vi "Drive Execute.vi"() -> ()   [LabVIEW 2017]
uses:
  Drive Control Type.ctl
  <vilib>/Rock Robotics/WPI/Solenoid/WPI_SolenoidValue.ctl
  <vilib>/Rock Robotics/WPI/DriverStation/WPI_DriverStationRobotMode2.ctl
  Drive Notifier.ctl
  <vilib>/Rock Robotics/WPI/ThirdParty/Phoenix-LabVIEW/Motor Controller/Controls/CTRE_Phoenix_MotorControl_ControlMode.ctl
  Drive Globals.vi
  Utility VIs/Refnum Names.vi
  Robot Global Data.vi
  <vilib>/Rock Robotics/WPI/Solenoid/WPI_SolenoidSetEnum.vi
  Autonomous/Autonomous Globals.vi
panel:
  out "Drive Motor Speeds-Teleop":T1(graph)
  out "error out":errorcluster
  in  "Maximum Low Linear Speed":dbl=5.49
  in  "Maximum High Linear Speed":dbl
  in  "Lower Multiplier":dbl=0.4
  in  "Upper Multiplier":dbl=0.65
  in  "Piecewise Turn Threshold":dbl=0.4
  in  "Lower Turn Speed":dbl=3.0
  in  "Upper Turn Speed":dbl=7.0
  in  "Scale Intertia":dbl=0.75
  # "Turning to Cube"
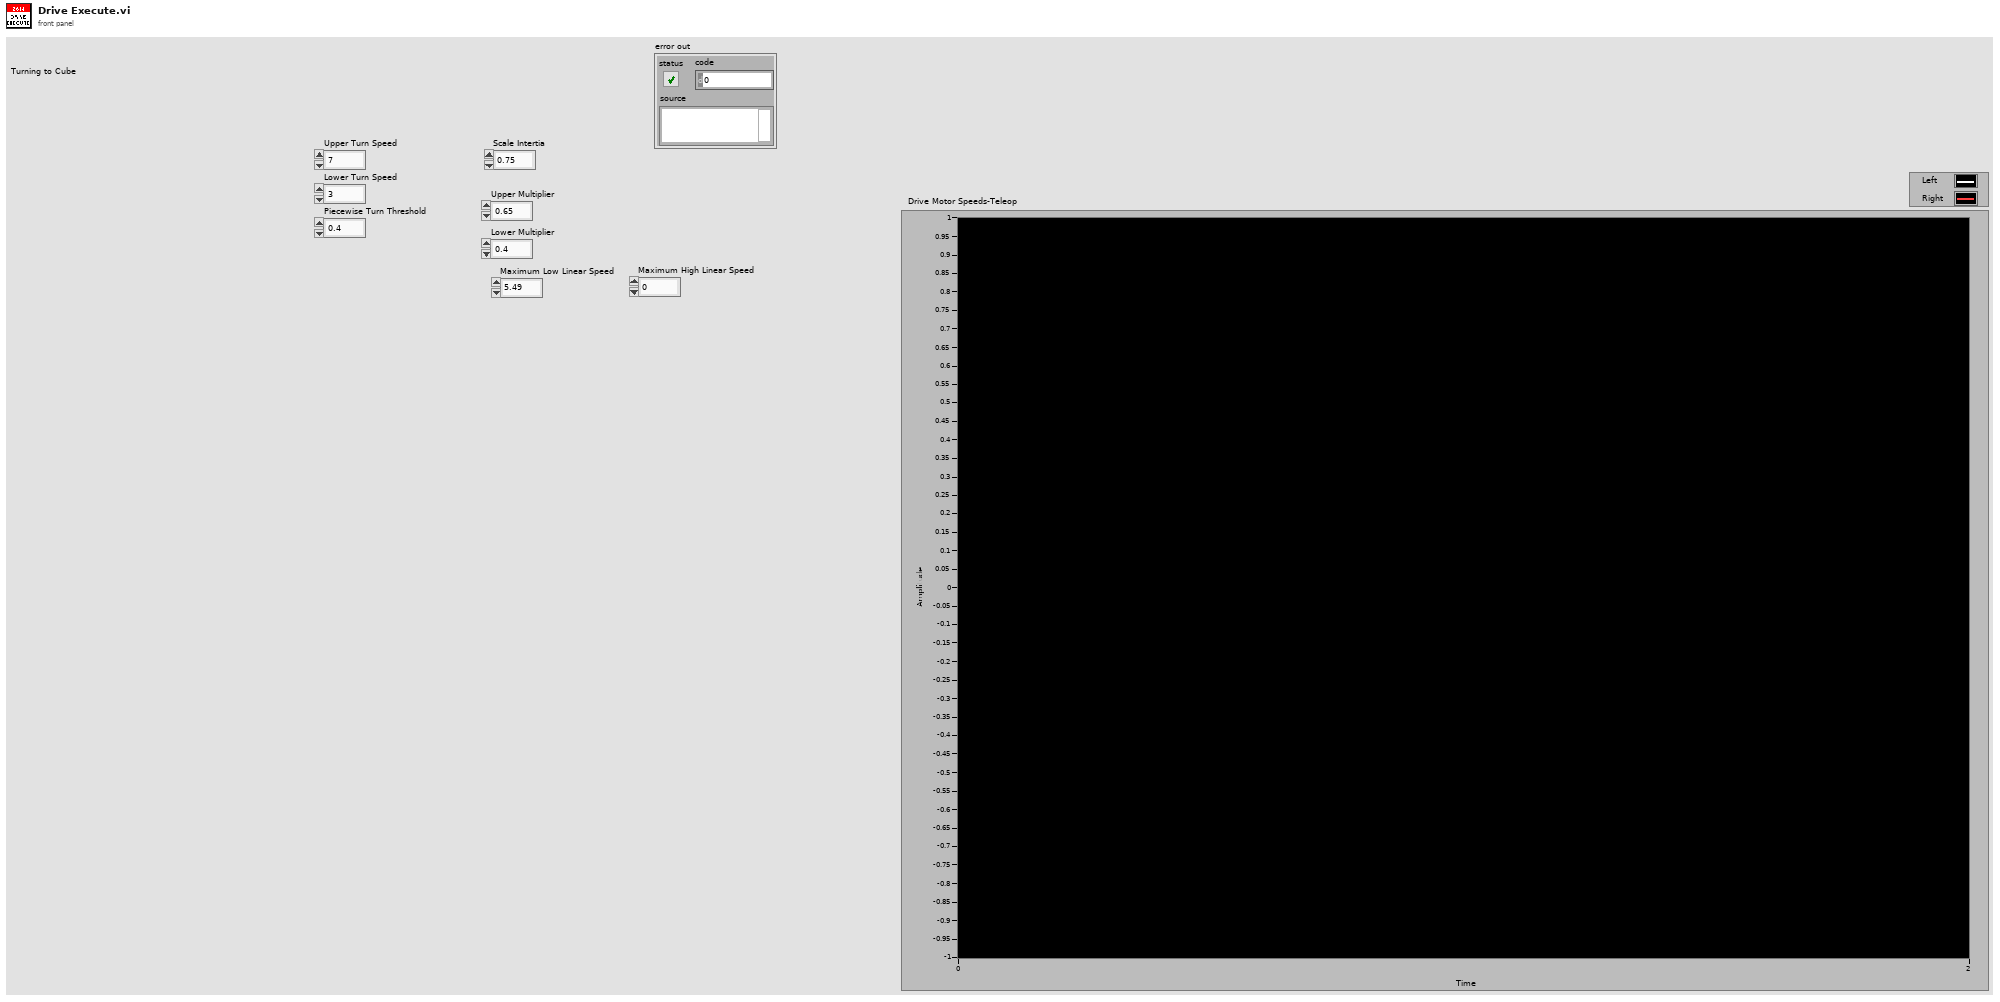
[diagram p1: front panel]
types:
  T1 = cluster{"Velocity (Raw Sensor Units per 100 ms)":i32, "Velocity (Raw Sensor Units per 100 ms)":i32, "Left Motor Value":dbl, dbl}
  T2 = typedef "WPI_MotorControlDeviceRef.ctl" = cluster{"DeviceStatus":errorcluster, "Type":T3, "PWM":cluster{"PWM Channel":T4, "DeadBand":T5}, "CAN":cluster{"Device Number":u8, "SetOutput VI Ref":variant, "GetOutput VI Ref":variant, "Enable VI Ref":variant, "Disable VI Ref":variant, "Data":variant}, "Invert":bool, "DIO PWM":cluster{"PWM \"Enable\" Channel":T4, "DIOChannel":T6, "PWM Rate":dbl}}
  T3 = typedef "WPI_MotorControlType.ctl" = enum16{"PWM", "CAN", "DIO PWM"}
  T4 = typedef "FPGA_DIOPWMChannel.ctl" = enum8{"PWM 0", "PWM 1", "PWM 2", "PWM 3", "PWM 4", "PWM 5", "PWM 6", "PWM 7", "PWM 8", "PWM 9", "PWM MXP 0", "PWM MXP 1", "PWM MXP 2", "PWM MXP 3", "PWM MXP 4", "PWM MXP 5", "PWM MXP 6", "PWM MXP 7", "PWM MXP 8", "PWM MXP 9", "Invalid"}
  T5 = typedef "WPI_PWMDeadband.ctl" = cluster{"Name":string, "maxPositivePwm":i32, "minPositivePwm":i32, "centerPwm":i32, "maxNegativePwm":i32, "minNegativePwm":i32, "angularRange":u16}
  T6 = typedef "FPGA_DIOChannel.ctl" = enum8{"DIO 0", "DIO 1", "DIO 2", "DIO 3", "DIO 4", "DIO 5", "DIO 6", "DIO 7", "DIO 8", "DIO 9", "DIO MXP 0", "DIO MXP 1", "DIO MXP 2", "DIO MXP 3", "DIO MXP 4", "DIO MXP 5", "DIO MXP 6", "DIO MXP 7", "DIO MXP 8", "DIO MXP 9", "DIO MXP 10", "DIO MXP 11", "DIO MXP 12", "DIO MXP 13", "DIO MXP 14", "DIO MXP 15", "SPI Port CS1", "SPI Port CS2", "SPI Port CS3", "SPI Port MISO", "SPI Port MOSI", "Invalid"}
  T7 = typedef "WPI_SolenoidDevRef.ctl" = cluster{"DevStatus":errorcluster, "Pneumatics Control Module":u8, "Forward Solenoid Channel":T8, "Reverse Solenoid Channel":T8}
  T8 = typedef "WPI_SolenoidChannel.ctl" = enum8{"Solenoid 0", "Solenoid 1", "Solenoid 2", "Solenoid 3", "Solenoid 4", "Solenoid 5", "Solenoid 6", "Solenoid 7", "Invalid"}
  T9 = typedef "WPI_SolenoidValue.ctl" = enum16{"Off", "On", "Forward", "Reverse"}
  T10 = typedef "Drive Control Type.ctl" = enum16{"No_Op", "Basic Drive", "Time", "Heading", "Hybrid_Turn", "RC_Speed", "Switch_Slots", "AutoTrack_Cube", "Speed Test", "Turn_Cube", "To_Cube", "Wait", "Distance_Slow", "Distance", "D_H_Delay", "Distance_Delay", "Heading_Cap", "Heading_Tight", "Cube_Heading", "Distance_Ramp"}
  T11 = typedef "WPI_DriverStationRobotMode2.ctl" = enum16{"Autonomous Disabled", "Autonomous Enabled", "Teleop Disabled", "Teleop Enabled", "Disconnected", "Finish", "Test Disabled", "Test Enabled", "Emergency Stopped"}
  T12 = typedef "Drive Notifier.ctl" = cluster{"Drive Control Type":T10, "Throttle":dbl, "Twist":dbl, "Step":i32, "High Gear":bool, "Parameter 1":dbl, "Parameter 2":dbl, "Parameter 3":dbl, "Drive Notifier":refnum<notifier>, "AutoTrack":bool}
  T13 = typedef "CTRE_Phoenix_MotorControl_ControlMode.ctl" = u16
  T14 = cluster{"offsetAngle H":dbl, "offsetAngle V":dbl, "area":dbl, "skew":dbl}
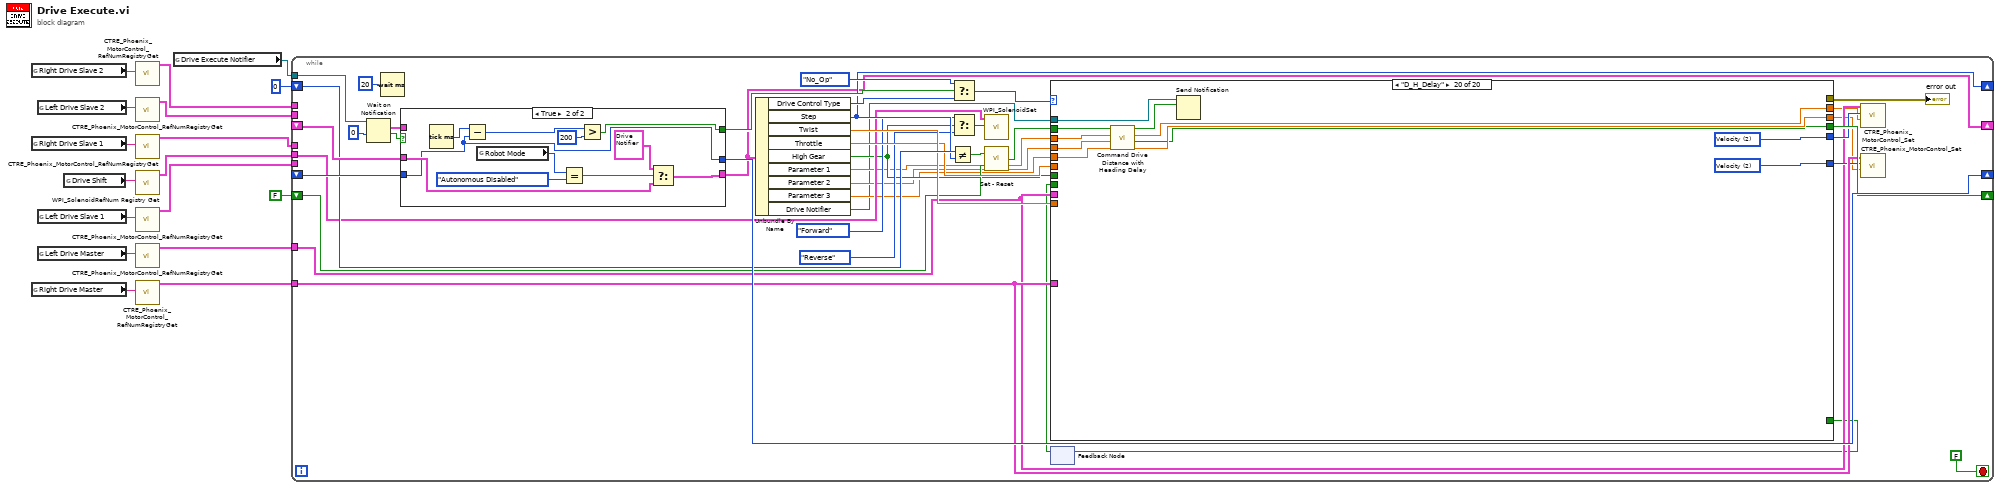
[diagram p0: block diagram]
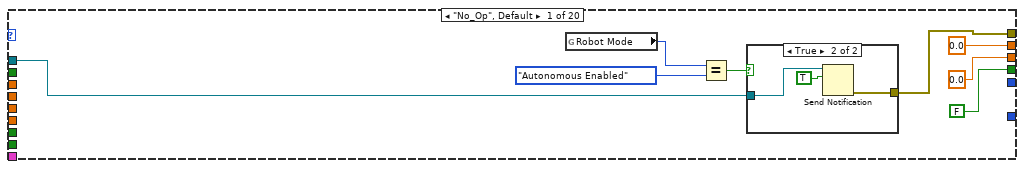
[diagram p2: hidden frame]
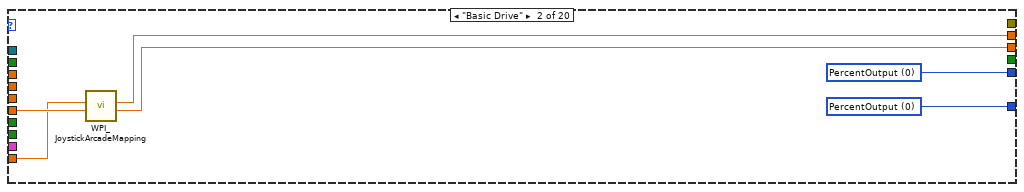
[diagram p4: hidden frame]
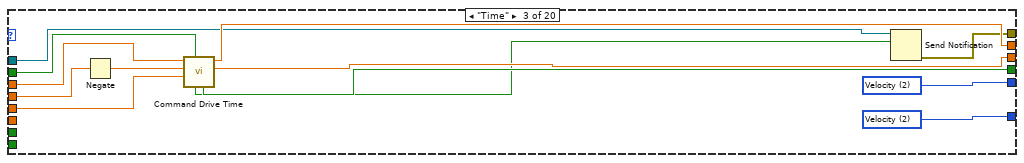
[diagram p5: hidden frame]
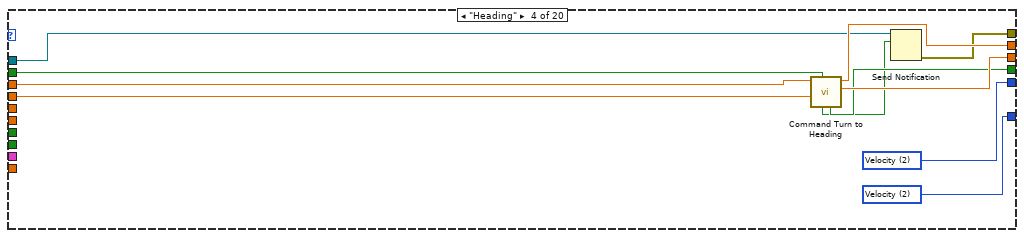
[diagram p6: hidden frame]
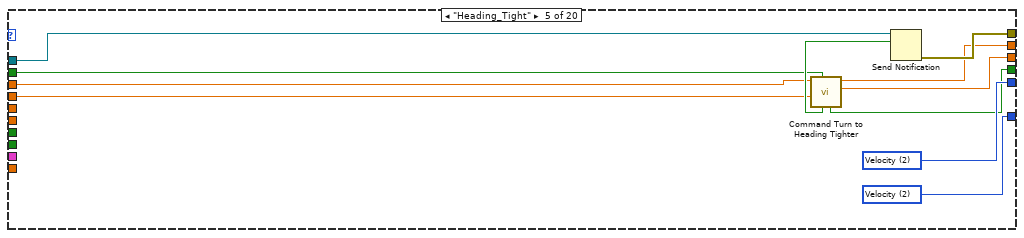
[diagram p7: hidden frame]
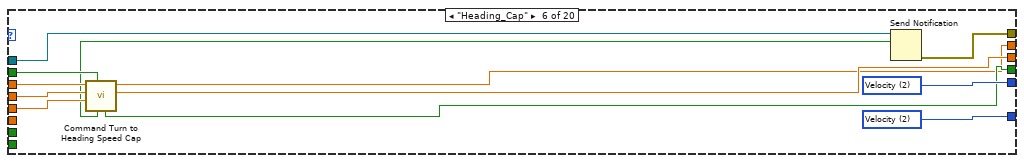
[diagram p8: hidden frame]
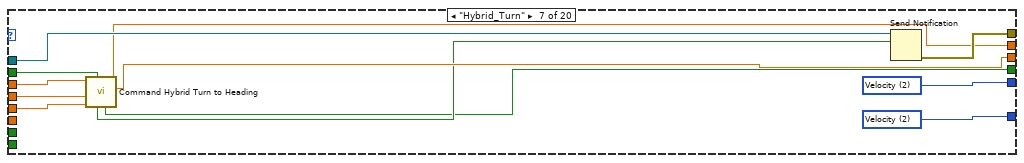
[diagram p9: hidden frame]
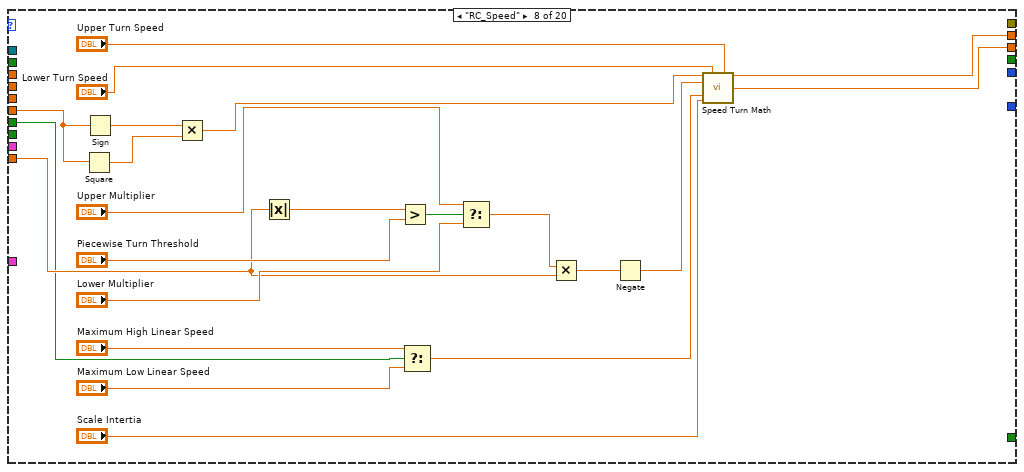
[diagram p10: hidden frame]
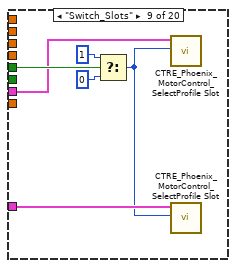
[diagram p11: hidden frame]
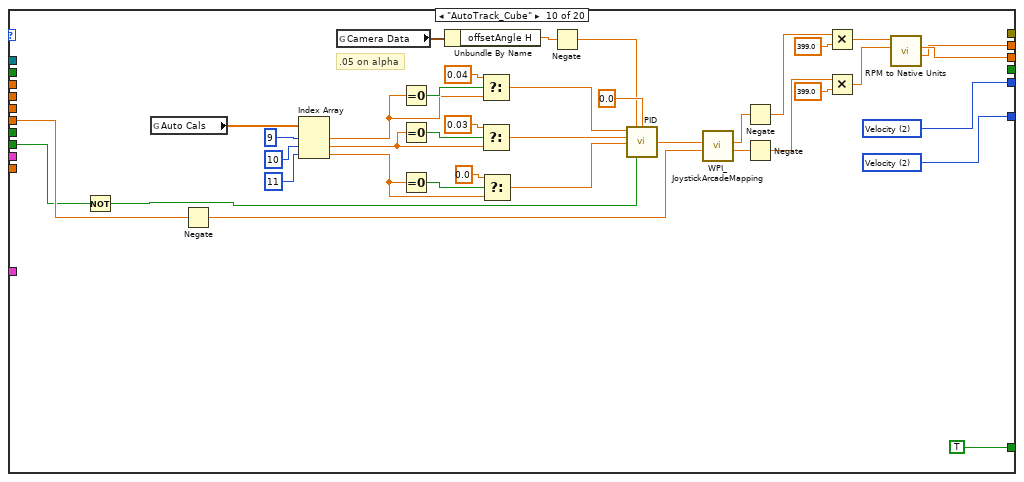
[diagram p12: hidden frame]
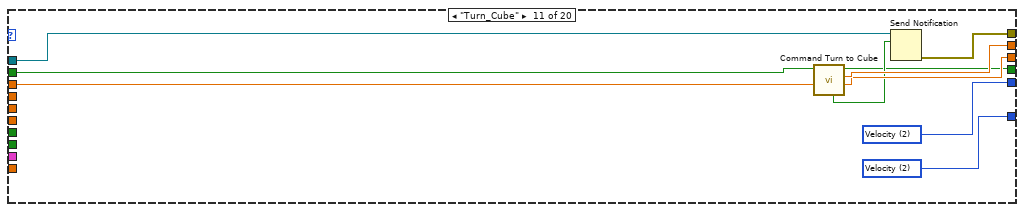
[diagram p13: hidden frame]
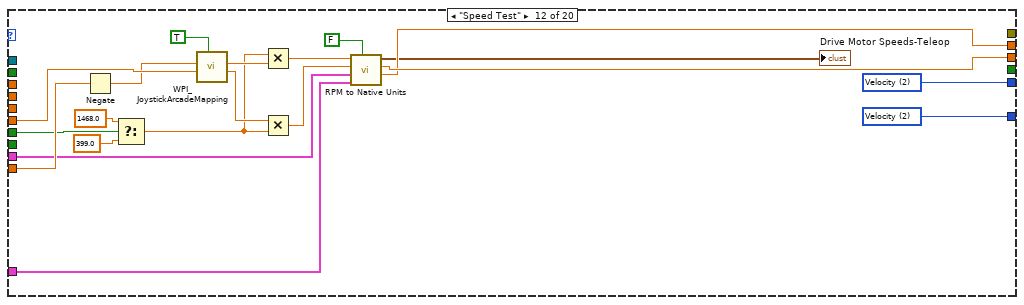
[diagram p14: hidden frame]
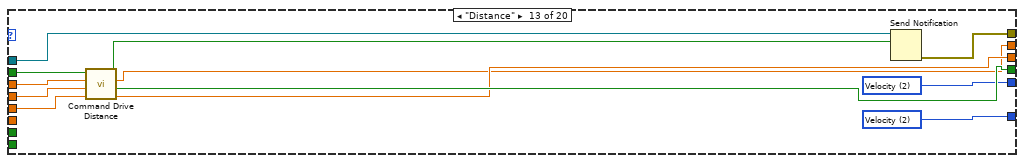
[diagram p15: hidden frame]
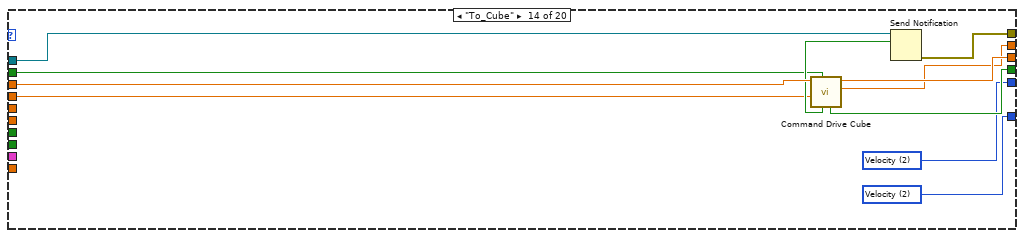
[diagram p16: hidden frame]
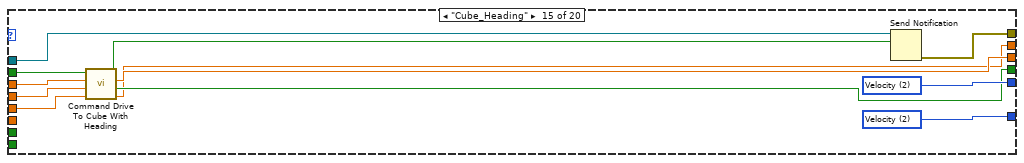
[diagram p17: hidden frame]
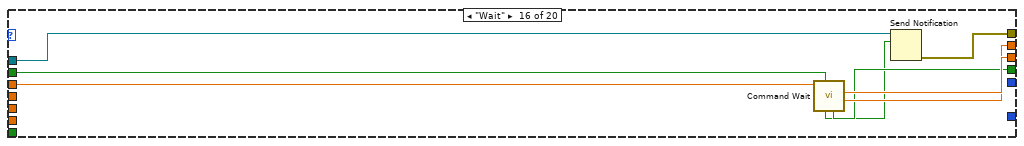
[diagram p18: hidden frame]
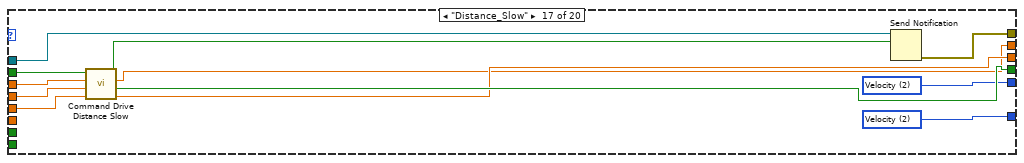
[diagram p19: hidden frame]
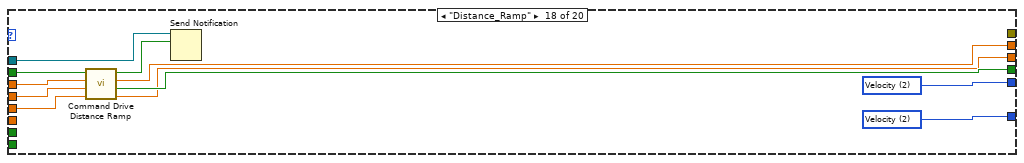
[diagram p20: hidden frame]
diagram:
  n1 = global read "Refnum Names.vi" "Right Drive Slave 2"() -> (w9:string)
  n2 = global read "Refnum Names.vi" "Right Drive Slave 1"() -> (w10:string)
  n3 = global read "Refnum Names.vi" "Right Drive Master"() -> (w16:string)
  n4 = global read "Refnum Names.vi" "Left Drive Slave 2"() -> (w7:string)
  n5 = global read "Refnum Names.vi" "Left Drive Slave 1"() -> (w8:string)
  n6 = global read "Refnum Names.vi" "Left Drive Master"() -> (w15:string)
  n7 = global read "Refnum Names.vi" "Drive Shift"() -> (w12:string)
  n8 = call <vilib>:"CTRE_Phoenix_MotorControl_RefNumRegistryGet.vi"("refnum name"=w9) -> ("PhoenixMotorControlDevRef"=w3:T2)  [unwired: 9 in, 1 out]
  n9 = call <vilib>:"CTRE_Phoenix_MotorControl_RefNumRegistryGet.vi"("refnum name"=w7) -> ("PhoenixMotorControlDevRef"=w4:T2)  [unwired: 9 in, 1 out]
  n10 = call <vilib>:"CTRE_Phoenix_MotorControl_RefNumRegistryGet.vi"("refnum name"=w10) -> ("PhoenixMotorControlDevRef"=w5:T2)  [unwired: 9 in, 1 out]
  n11 = call <vilib>:"WPI_SolenoidRefNum Registry Get.vi"("refnum name"=w12) -> ("SolenoidDevRef"=w11:T7)  [unwired: 9 in, 1 out]
  n12 = call <vilib>:"CTRE_Phoenix_MotorControl_RefNumRegistryGet.vi"("refnum name"=w8) -> ("PhoenixMotorControlDevRef"=w6:T2)  [unwired: 9 in, 1 out]
  n13 = call <vilib>:"CTRE_Phoenix_MotorControl_RefNumRegistryGet.vi"("refnum name"=w15) -> ("PhoenixMotorControlDevRef"=w14:T2)  [unwired: 9 in, 1 out]
  n14 = call <vilib>:"CTRE_Phoenix_MotorControl_RefNumRegistryGet.vi"("refnum name"=w16) -> ("PhoenixMotorControlDevRef"=w13:T2)  [unwired: 9 in, 1 out]
  n15 = global read "Drive Globals.vi" "Drive Execute Notifier"() -> (w17:refnum<notifier>)
  n16 = while {
    tunnel: w17 -> [w55]
    shift-right: [w29] -> _
    shift-left: _ -> [w52]
    shift-right: [w50] -> _
    shift-left: _ -> [w49]
    shift-right: [w43] -> _
    shift-left: 0 ("Step") -> [w44]
    tunnel: w14 -> [w28]
    tunnel: w13 -> [w33]
    tunnel: w11 -> [w40]
    shift-right: [w35] -> _
    shift-left: FALSE ("Output") -> [w34]
    tunnel: w4 -> [_]
    tunnel: w6 -> [_]
    tunnel: w5 -> [_]
    tunnel: w3 -> [_]
    stop <- FALSE stop-if-true
    n17 = Wait on Notification(notifier=w55, timeout in ms (-1)=0) -> (notification=w51:T12, timed out?=w53:bool)  [unwired: 2 in, 2 out]
    n18 = Wait (ms)(milliseconds to wait=u32 20) -> ()  [unwired: 1 out]
    n19 = case shown="True" w53 {
      tunnel: w52 -> [_ w330]
      tunnel: [w320 w329] -> w29
      tunnel: w51 -> [w320 _]
      tunnel: [w319 w322] -> w50
      tunnel: w49 -> [_ w322]
      tunnel: [FALSE w325] -> w46
      frame False {
        n20 = Tick Count (ms)() -> (millisecond timer value=w319:u32)
      }
      frame True {
        n21 = Tick Count (ms)() -> (millisecond timer value=w328:u32)
        n22 = Subtract(x=w328, y=w322) -> (x-y=w327:u32)
        n23 = global read "Robot Global Data.vi" "Robot Mode"() -> (w324:T11)
        n24 = Equal?(x=w324, y=WPI_DriverStationRobotMode2."Autonomous Disabled") -> (x = y?=w331:bool)
        n25 = Greater?(x=w327, y=u32 200) -> (0:w325:bool)
        n26 = Select(t=T12 {"Drive Control Type"=enum."No_Op", "Throttle"=0.0, "Twist"=0.0, "Step"=0, "High Gear"=FALSE, "Parameter 1"=0.0, "Parameter 2"=0.0, "Parameter 3"=0.0, "Drive Notifier"=refnum, "AutoTrack"=FALSE} ("Drive Notifier"), s=w331, f=w330) -> (s? t:f=w329:T12)
      }
    }
    n27 = Unbundle By Name(w29) -> ("Drive Control Type"=w48:T10, "Step"=w43:i32, "Twist"=w42:dbl, "Throttle"=w41:dbl, "High Gear"=w32:bool, "Parameter 1"=w26:dbl, "Parameter 2"=w25:dbl, "Parameter 3"=w24:dbl, "Drive Notifier"=w23:refnum<notifier>)
    n28 = Not Equal?(x=w44, y=w43) -> (x != y?=w27:bool)
    n29 = Select(t=Drive_Control_Type."No_Op", s=w46, f=w48) -> (s? t:f=w47:T10)
    n30 = Select(t=WPI_SolenoidValue."Forward" ("Value"), s=w32, f=WPI_SolenoidValue."Reverse" ("Value")) -> (s? t:f=w37:T9)
    n31 = call-poly <vilib>:"WPI_SolenoidSet.vi"("Value"=w37, "SolenoidDevRef"=w40) -> ()  [unwired: 8 in, 2 out]
    n32 = call "Set - Reset.vi"("Reset"=w34, "Set"=w27) -> ("Output"=w36:bool)
    n33 = feedback #1() -> (w19:bool)  [unwired: 1 in]
    n34 = case shown="\"D_H_Delay\"" w47 {
      tunnel: w42 -> [_ w72 _ _ _ _ _ w140 _ _ _ w228 _ _ _ _ _ _ _ _]
      tunnel: w41 -> [_ w73 _ _ _ _ _ w141 _ w194 _ w229 _ _ _ _ _ _ _ _]
      tunnel: [0.0 ("Left Motor Value") w70 w84 w96 w100 w110 w128 w139 _ w181 w209 w214 w235 w244 w253 w269 w275 w285 w303 w309] -> w21
      tunnel: [0.0 ("Right Motor Value") w69 w83 w95 w99 w111 w127 w138 _ w182 w208 w215 w236 w245 w254 w270 w276 w286 w302 w308] -> w22
      tunnel: [_ w71 w77 w90 w107 w119 w131 _ _ w196 w206 w224 w233 w247 w263 _ w274 w295 w306 w317] -> w31
      tunnel: [_ w74 w76 w91 w108 w120 w132 _ _ w197 w207 w223 w234 w246 w262 _ w273 w294 w305 w316] -> w30
      tunnel: w36 -> [_ _ w82 w98 w103 w114 w129 _ _ _ w205 _ w241 w248 w257 w272 w284 w290 w296 w311]
      tunnel: [FALSE ("Reint") _ w81 w94 w104 w112 w125 _ _ _ w202 _ w240 w249 w255 w268 w277 w287 w300 w307] -> w35
      tunnel: w33 -> [_ _ _ _ _ _ _ _ w161 _ _ w211 _ _ _ _ _ _ _ _]
      tunnel: w32 -> [_ _ _ _ _ _ _ w136 w160 _ _ w219 _ _ _ _ _ _ _ _]
      tunnel: w28 -> [_ _ _ _ _ _ _ _ w156 _ _ w212 _ _ _ _ _ _ _ _]
      tunnel: w26 -> [_ _ w87 w97 w102 w115 w124 _ _ _ w201 _ w239 w252 w258 w271 w283 w291 w297 w312]
      tunnel: w25 -> [_ _ w86 w89 w101 w117 w123 _ _ _ _ _ w232 w243 w259 _ w282 w292 w298 w313]
      tunnel: w24 -> [_ _ w85 _ _ w116 w122 _ _ _ _ _ w231 _ w260 _ w281 w293 w299 w314]
      tunnel: w23 -> [w61 _ w80 w93 w109 w121 w133 _ _ _ w203 _ w237 w250 w264 w266 w280 w289 w304 w315]
      tunnel: [w59 _ w75 w88 w106 w118 w130 _ _ _ w200 _ w230 w242 w261 w265 w279 _ _ _] -> w20
      tunnel: w19 -> [_ _ _ _ _ _ _ _ _ w164 _ _ _ _ _ _ _ _ _ _]
      tunnel: [_ _ _ _ _ _ _ _ _ TRUE _ _ _ _ _ _ _ _ _ _] -> w18
      frame "No_Op", Default {
        n35 = global read "Robot Global Data.vi" "Robot Mode"() -> (w60:T11)
        n36 = Equal?(x=w60, y=WPI_DriverStationRobotMode2."Autonomous Enabled") -> (x = y?=w62:bool)
        n37 = case shown="True" w62 {
          tunnel: w61 -> [_ w68]
          tunnel: [_ w66] -> w59
          frame False {
          }
          frame True {
            n38 = Send Notification(notification=TRUE, notifier=w68) -> (error out=w66:errorcluster)  [unwired: 1 in, 1 out]
          }
        }
      }
      frame "Basic Drive" {
        w74 = T13 0 items=["PercentOutput"=0, "Position"=1, "Velocity"=2, "Current"=3, "Follower"=5, "MotionProfile"=6, "MotionMagic"=7, "MotionMagicArc"=8, "MotionProfileArc"=10, "Disabled"=15] ("Control Mode")
        w71 = T13 0 items=["PercentOutput"=0, "Position"=1, "Velocity"=2, "Current"=3, "Follower"=5, "MotionProfile"=6, "MotionMagic"=7, "MotionMagicArc"=8, "MotionProfileArc"=10, "Disabled"=15] ("Control Mode")
        n39 = call <vilib>:"WPI_JoystickArcadeMapping.vi"("Y axis value"=w73, "X axis value"=w72) -> ("Right Motor Value"=w69:dbl, "Left Motor Value"=w70:dbl)  [unwired: 8 in]
      }
      frame "Time" {
        w76 = T13 2 items=["PercentOutput"=0, "Position"=1, "Velocity"=2, "Current"=3, "Follower"=5, "MotionProfile"=6, "MotionMagic"=7, "MotionMagicArc"=8, "MotionProfileArc"=10, "Disabled"=15] ("Control Mode")
        w77 = T13 2 items=["PercentOutput"=0, "Position"=1, "Velocity"=2, "Current"=3, "Follower"=5, "MotionProfile"=6, "MotionMagic"=7, "MotionMagicArc"=8, "MotionProfileArc"=10, "Disabled"=15] ("Control Mode")
        n40 = Negate(x=w86) -> (-x=w78:dbl)
        n41 = call "Command Drive Time.vi"("Startup"=w82, "Translation (Throttle)"=w85, "Drive (Throttle)"=w78, "Time to Run (ms)"=w87) -> ("Right Wheel"=w83:dbl, "Left Wheel"=w84:dbl, "Reinit"=w81:bool, "Completed"=w79:bool)  [unwired: 4 in]
        n42 = Send Notification(notification=w79, notifier=w80) -> (error out=w75:errorcluster)  [unwired: 1 in, 1 out]
      }
      frame "Heading" {
        w90 = T13 2 items=["PercentOutput"=0, "Position"=1, "Velocity"=2, "Current"=3, "Follower"=5, "MotionProfile"=6, "MotionMagic"=7, "MotionMagicArc"=8, "MotionProfileArc"=10, "Disabled"=15] ("Control Mode")
        w91 = T13 2 items=["PercentOutput"=0, "Position"=1, "Velocity"=2, "Current"=3, "Follower"=5, "MotionProfile"=6, "MotionMagic"=7, "MotionMagicArc"=8, "MotionProfileArc"=10, "Disabled"=15] ("Control Mode")
        n43 = call "Command Turn to Heading.vi"("Startup"=w98, "Timeout"=w89, "Heading"=w97) -> ("Right Wheel Velocity"=w95:dbl, "Left Wheel Velocity"=w96:dbl, "Reint"=w94:bool, "Completed"=w92:bool)  [unwired: 5 in]
        n44 = Send Notification(notification=w92, notifier=w93) -> (error out=w88:errorcluster)  [unwired: 1 in, 1 out]
      }
      frame "Heading_Tight" {
        w107 = T13 2 items=["PercentOutput"=0, "Position"=1, "Velocity"=2, "Current"=3, "Follower"=5, "MotionProfile"=6, "MotionMagic"=7, "MotionMagicArc"=8, "MotionProfileArc"=10, "Disabled"=15] ("Control Mode")
        w108 = T13 2 items=["PercentOutput"=0, "Position"=1, "Velocity"=2, "Current"=3, "Follower"=5, "MotionProfile"=6, "MotionMagic"=7, "MotionMagicArc"=8, "MotionProfileArc"=10, "Disabled"=15] ("Control Mode")
        n45 = call "Command Turn to Heading Tighter.vi"("Startup"=w103, "Timeout"=w101, "Heading"=w102) -> ("Right Wheel Velocity"=w99:dbl, "Left Wheel Velocity"=w100:dbl, "Reint"=w104:bool, "Completed"=w105:bool)  [unwired: 5 in]
        n46 = Send Notification(notification=w105, notifier=w109) -> (error out=w106:errorcluster)  [unwired: 1 in, 1 out]
      }
      frame "Heading_Cap" {
        w119 = T13 2 items=["PercentOutput"=0, "Position"=1, "Velocity"=2, "Current"=3, "Follower"=5, "MotionProfile"=6, "MotionMagic"=7, "MotionMagicArc"=8, "MotionProfileArc"=10, "Disabled"=15] ("Control Mode")
        w120 = T13 2 items=["PercentOutput"=0, "Position"=1, "Velocity"=2, "Current"=3, "Follower"=5, "MotionProfile"=6, "MotionMagic"=7, "MotionMagicArc"=8, "MotionProfileArc"=10, "Disabled"=15] ("Control Mode")
        n47 = call "Command Turn to Heading Speed Cap.vi"("Startup"=w114, "Timeout"=w116, "Max Speed"=w117, "Heading"=w115) -> ("Right Wheel Velocity"=w111:dbl, "Left Wheel Velocity"=w110:dbl, "Reint"=w112:bool, "Completed"=w113:bool)  [unwired: 4 in]
        n48 = Send Notification(notification=w113, notifier=w121) -> (error out=w118:errorcluster)  [unwired: 1 in, 1 out]
      }
      frame "Hybrid_Turn" {
        w131 = T13 2 items=["PercentOutput"=0, "Position"=1, "Velocity"=2, "Current"=3, "Follower"=5, "MotionProfile"=6, "MotionMagic"=7, "MotionMagicArc"=8, "MotionProfileArc"=10, "Disabled"=15] ("Control Mode")
        w132 = T13 2 items=["PercentOutput"=0, "Position"=1, "Velocity"=2, "Current"=3, "Follower"=5, "MotionProfile"=6, "MotionMagic"=7, "MotionMagicArc"=8, "MotionProfileArc"=10, "Disabled"=15] ("Control Mode")
        n49 = call "Command Hybrid Turn to Heading.vi"("Startup"=w129, "Timeout"=w122, "Translation (Throttle)"=w123, "Heading"=w124) -> ("Right Wheel"=w127:dbl, "Left Wheel"=w128:dbl, "Reinit"=w125:bool, "Completed"=w126:bool)  [unwired: 4 in]
        n50 = Send Notification(notification=w126, notifier=w133) -> (error out=w130:errorcluster)  [unwired: 1 in, 1 out]
      }
      frame "RC_Speed" {
        n51 = Square(x=w141) -> (x^2=w155:dbl)
        n52 = Sign(1:w141) -> (0:w154:dbl)
        n53 = Multiply(x=w154, y=w155) -> (x*y=w153:dbl)
        n54 = Absolute Value(x=w140) -> (abs(x)=w148:dbl)
        n55 = Greater?(x=w148, y="Piecewise Turn Threshold") -> (0:w147:bool)
        n56 = Select(t="Maximum High Linear Speed", s=w136, f="Maximum Low Linear Speed") -> (s? t:f=w137:dbl)
        n57 = Select(t="Upper Multiplier", s=w147, f="Lower Multiplier") -> (s? t:f=w145:dbl)
        n58 = Multiply(x=w145, y=w140) -> (x*y=w144:dbl)
        n59 = Negate(x=w144) -> (-x=w151:dbl)
        n60 = call "Speed Turn Math.vi"("Throttle"=w153, "Lower Turn Speed"="Lower Turn Speed", "Upper Turn Speed"="Upper Turn Speed", "Turn"=w151, "Maximum Linear Speed"=w137, "Scale Intertia"="Scale Intertia") -> ("Left Wheel Velocity"=w139:dbl, "Right Wheel Velocity"=w138:dbl)  [unwired: 8 in]
      }
      frame "Switch_Slots" {
        n61 = Select(t=1, s=w160, f=0) -> (s? t:f=w157:i32)
        n62 = call <vilib>:"CTRE_Phoenix_MotorControl_SelectProfile Slot.vi"("slotIdx"=w157, "PhoenixMotorControlDevRef"=w156) -> ()  [unwired: 8 in, 2 out]
        n63 = call <vilib>:"CTRE_Phoenix_MotorControl_SelectProfile Slot.vi"("slotIdx"=w157, "PhoenixMotorControlDevRef"=w161) -> ()  [unwired: 8 in, 2 out]
      }
      frame "AutoTrack_Cube" {
        w196 = T13 2 items=["PercentOutput"=0, "Position"=1, "Velocity"=2, "Current"=3, "Follower"=5, "MotionProfile"=6, "MotionMagic"=7, "MotionMagicArc"=8, "MotionProfileArc"=10, "Disabled"=15] ("Control Mode")
        w197 = T13 2 items=["PercentOutput"=0, "Position"=1, "Velocity"=2, "Current"=3, "Follower"=5, "MotionProfile"=6, "MotionMagic"=7, "MotionMagicArc"=8, "MotionProfileArc"=10, "Disabled"=15] ("Control Mode")
        # ".05 on alpha"
        n64 = Not(x=w164) -> (.not. x?=w162:bool)
        n65 = global read "Autonomous Globals.vi" "Auto Cals"() -> (w180:dbl[])
        n66 = Negate(x=w194) -> (-x=w192:dbl)
        n67 = Index Array(array=w180, index #1=9 ("index"), index #2=10 ("index"), index #3=11 ("index")) -> (element #1=w175:dbl, element #2=w171:dbl, element #3=w168:dbl)
        n68 = global read "Robot Global Data.vi" "Camera Data"() -> (w199:T14)
        n69 = Equal To 0?(x=w175) -> (x = 0?=w176:bool)
        n70 = Equal To 0?(x=w171) -> (x = 0?=w172:bool)
        n71 = Equal To 0?(x=w168) -> (x = 0?=w170:bool)
        n72 = Unbundle By Name(w199) -> ("offsetAngle H"=w195:dbl)
        n73 = Select(t=0.04, s=w176, f=w175) -> (s? t:f=w167:dbl)
        n74 = Select(t=0.03, s=w172, f=w171) -> (s? t:f=w166:dbl)
        n75 = Select(t=0.0, s=w170, f=w168) -> (s? t:f=w165:dbl)
        n76 = Negate(x=w195) -> (-x=w185:dbl)
        n77 = call "PID.vi"("Kp"=w167, "Process Variable"=w185, "Goal"=0.0, "Ki"=w166, "Kd"=w165, "Reinit"=w162) -> ("Command"=w193:dbl)  [unwired: 7 in, 2 out]
        n78 = call <vilib>:"WPI_JoystickArcadeMapping.vi"("Y axis value"=w192, "X axis value"=w193) -> ("Right Motor Value"=w190:dbl, "Left Motor Value"=w191:dbl)  [unwired: 8 in]
        n79 = Negate(x=w191) -> (-x=w189:dbl)
        n80 = Negate(x=w190) -> (-x=w188:dbl)
        n81 = Multiply(x=w189, y=399.0) -> (x*y=w184:dbl)
        n82 = Multiply(x=w188, y=399.0) -> (x*y=w183:dbl)
        n83 = call "RPM to Native Units.vi"("Right RPM"=w183, "Left RPM"=w184) -> ("Right Out"=w181:dbl, "Left Out"=w182:dbl)  [unwired: 6 in, 1 out]
      }
      frame "Turn_Cube" {
        w206 = T13 2 items=["PercentOutput"=0, "Position"=1, "Velocity"=2, "Current"=3, "Follower"=5, "MotionProfile"=6, "MotionMagic"=7, "MotionMagicArc"=8, "MotionProfileArc"=10, "Disabled"=15] ("Control Mode")
        w207 = T13 2 items=["PercentOutput"=0, "Position"=1, "Velocity"=2, "Current"=3, "Follower"=5, "MotionProfile"=6, "MotionMagic"=7, "MotionMagicArc"=8, "MotionProfileArc"=10, "Disabled"=15] ("Control Mode")
        n84 = call "Command Turn to Cube.vi"("Timeout"=w201, "Startup"=w205) -> ("Right Wheel Velocity"=w208:dbl, "Left Wheel Velocity"=w209:dbl, "Reint"=w202:bool, "Completed"=w204:bool)  [unwired: 6 in]
        n85 = Send Notification(notification=w204, notifier=w203) -> (error out=w200:errorcluster)  [unwired: 1 in, 1 out]
      }
      frame "Speed Test" {
        w223 = T13 2 items=["PercentOutput"=0, "Position"=1, "Velocity"=2, "Current"=3, "Follower"=5, "MotionProfile"=6, "MotionMagic"=7, "MotionMagicArc"=8, "MotionProfileArc"=10, "Disabled"=15] ("Control Mode")
        w224 = T13 2 items=["PercentOutput"=0, "Position"=1, "Velocity"=2, "Current"=3, "Follower"=5, "MotionProfile"=6, "MotionMagic"=7, "MotionMagicArc"=8, "MotionProfileArc"=10, "Disabled"=15] ("Control Mode")
        n86 = Negate(x=w228) -> (-x=w218:dbl)
        n87 = Select(t=1468.0, s=w219, f=399.0 ("y")) -> (s? t:f=w221:dbl)
        n88 = call <vilib>:"WPI_JoystickArcadeMapping.vi"("Square Inputs"=TRUE, "Y axis value"=w229, "X axis value"=w218) -> ("Right Motor Value"=w227:dbl, "Left Motor Value"=w225:dbl)  [unwired: 7 in]
        n89 = Multiply(x=w221, y=w225) -> (x*y=w217:dbl)
        n90 = Multiply(x=w227, y=w221) -> (x*y=w216:dbl)
        n91 = call "RPM to Native Units.vi"("Graph"=FALSE, "Right Talon"=w211, "Left Talon"=w212, "Right RPM"=w216, "Left RPM"=w217) -> ("Right Out"=w214:dbl, "Left Out"=w215:dbl, "Speeds"=→"Drive Motor Speeds-Teleop":T1)  [unwired: 3 in]
      }
      frame "Distance" {
        w233 = T13 2 items=["PercentOutput"=0, "Position"=1, "Velocity"=2, "Current"=3, "Follower"=5, "MotionProfile"=6, "MotionMagic"=7, "MotionMagicArc"=8, "MotionProfileArc"=10, "Disabled"=15] ("Control Mode")
        w234 = T13 2 items=["PercentOutput"=0, "Position"=1, "Velocity"=2, "Current"=3, "Follower"=5, "MotionProfile"=6, "MotionMagic"=7, "MotionMagicArc"=8, "MotionProfileArc"=10, "Disabled"=15] ("Control Mode")
        n92 = call "Command Drive Distance.vi"("Timeout"=w231, "Heading"=w232, "Distance"=w239, "Startup"=w241) -> ("Right Wheel"=w236:dbl, "Reinit"=w240:bool, "Left Wheel"=w235:dbl, "Completed"=w238:bool)  [unwired: 4 in]
        n93 = Send Notification(notification=w238, notifier=w237) -> (error out=w230:errorcluster)  [unwired: 1 in, 1 out]
      }
      frame "To_Cube" {
        w246 = T13 2 items=["PercentOutput"=0, "Position"=1, "Velocity"=2, "Current"=3, "Follower"=5, "MotionProfile"=6, "MotionMagic"=7, "MotionMagicArc"=8, "MotionProfileArc"=10, "Disabled"=15] ("Control Mode")
        w247 = T13 2 items=["PercentOutput"=0, "Position"=1, "Velocity"=2, "Current"=3, "Follower"=5, "MotionProfile"=6, "MotionMagic"=7, "MotionMagicArc"=8, "MotionProfileArc"=10, "Disabled"=15] ("Control Mode")
        n94 = call "Command Drive Cube.vi"("Startup"=w248, "Timeout"=w243, "Speed"=w252) -> ("Right Wheel"=w244:dbl, "Left Wheel"=w245:dbl, "Reinit"=w249:bool, "Completed"=w251:bool)  [unwired: 5 in]
        n95 = Send Notification(notification=w251, notifier=w250) -> (error out=w242:errorcluster)  [unwired: 1 in, 1 out]
      }
      frame "Cube_Heading" {
        w262 = T13 2 items=["PercentOutput"=0, "Position"=1, "Velocity"=2, "Current"=3, "Follower"=5, "MotionProfile"=6, "MotionMagic"=7, "MotionMagicArc"=8, "MotionProfileArc"=10, "Disabled"=15] ("Control Mode")
        w263 = T13 2 items=["PercentOutput"=0, "Position"=1, "Velocity"=2, "Current"=3, "Follower"=5, "MotionProfile"=6, "MotionMagic"=7, "MotionMagicArc"=8, "MotionProfileArc"=10, "Disabled"=15] ("Control Mode")
        n96 = call "Command Drive To Cube With Heading.vi"("Timeout"=w260, "Heading"=w259, "Speed"=w258, "Startup"=w257) -> ("Right Wheel"=w253:dbl, "Reinit"=w255:bool, "Left Wheel"=w254:dbl, "Completed"=w256:bool)  [unwired: 4 in]
        n97 = Send Notification(notification=w256, notifier=w264) -> (error out=w261:errorcluster)  [unwired: 1 in, 1 out]
      }
      frame "Wait" {
        n98 = call "Command Wait.vi"("Startup"=w272, "Time to Wait (ms)"=w271) -> ("Right Wheel"=w269:dbl, "Left Wheel"=w270:dbl, "Reint"=w268:bool, "Completed"=w267:bool)  [unwired: 6 in]
        n99 = Send Notification(notification=w267, notifier=w266) -> (error out=w265:errorcluster)  [unwired: 1 in, 1 out]
      }
      frame "Distance_Slow" {
        w273 = T13 2 items=["PercentOutput"=0, "Position"=1, "Velocity"=2, "Current"=3, "Follower"=5, "MotionProfile"=6, "MotionMagic"=7, "MotionMagicArc"=8, "MotionProfileArc"=10, "Disabled"=15] ("Control Mode")
        w274 = T13 2 items=["PercentOutput"=0, "Position"=1, "Velocity"=2, "Current"=3, "Follower"=5, "MotionProfile"=6, "MotionMagic"=7, "MotionMagicArc"=8, "MotionProfileArc"=10, "Disabled"=15] ("Control Mode")
        n100 = call "Command Drive Distance Slow.vi"("Timeout"=w281, "Heading"=w282, "Distance"=w283, "Startup"=w284) -> ("Right Wheel"=w276:dbl, "Reinit"=w277:bool, "Left Wheel"=w275:dbl, "Completed"=w278:bool)  [unwired: 4 in]
        n101 = Send Notification(notification=w278, notifier=w280) -> (error out=w279:errorcluster)  [unwired: 1 in, 1 out]
      }
      frame "Distance_Ramp" {
        w294 = T13 2 items=["PercentOutput"=0, "Position"=1, "Velocity"=2, "Current"=3, "Follower"=5, "MotionProfile"=6, "MotionMagic"=7, "MotionMagicArc"=8, "MotionProfileArc"=10, "Disabled"=15] ("Control Mode")
        w295 = T13 2 items=["PercentOutput"=0, "Position"=1, "Velocity"=2, "Current"=3, "Follower"=5, "MotionProfile"=6, "MotionMagic"=7, "MotionMagicArc"=8, "MotionProfileArc"=10, "Disabled"=15] ("Control Mode")
        n102 = call "Command Drive Distance Ramp.vi"("Ramp_Distance"=w293, "Heading"=w292, "Distance"=w291, "Startup"=w290) -> ("Right Wheel"=w286:dbl, "Reinit"=w287:bool, "Left Wheel"=w285:dbl, "Completed"=w288:bool)  [unwired: 4 in]
        n103 = Send Notification(notification=w288, notifier=w289) -> ()  [unwired: 1 in, 2 out]
      }
      frame "Distance_Delay" {
        w305 = T13 2 items=["PercentOutput"=0, "Position"=1, "Velocity"=2, "Current"=3, "Follower"=5, "MotionProfile"=6, "MotionMagic"=7, "MotionMagicArc"=8, "MotionProfileArc"=10, "Disabled"=15] ("Control Mode")
        w306 = T13 2 items=["PercentOutput"=0, "Position"=1, "Velocity"=2, "Current"=3, "Follower"=5, "MotionProfile"=6, "MotionMagic"=7, "MotionMagicArc"=8, "MotionProfileArc"=10, "Disabled"=15] ("Control Mode")
        n104 = call "Command Drive Distance Delay.vi"("Turn_Distance"=w299, "Heading"=w298, "Distance"=w297, "Startup"=w296) -> ("Right Wheel"=w302:dbl, "Reinit"=w300:bool, "Left Wheel"=w303:dbl, "Completed"=w301:bool)  [unwired: 4 in]
        n105 = Send Notification(notification=w301, notifier=w304) -> ()  [unwired: 1 in, 2 out]
      }
      frame "D_H_Delay" {
        w316 = T13 2 items=["PercentOutput"=0, "Position"=1, "Velocity"=2, "Current"=3, "Follower"=5, "MotionProfile"=6, "MotionMagic"=7, "MotionMagicArc"=8, "MotionProfileArc"=10, "Disabled"=15] ("Control Mode")
        w317 = T13 2 items=["PercentOutput"=0, "Position"=1, "Velocity"=2, "Current"=3, "Follower"=5, "MotionProfile"=6, "MotionMagic"=7, "MotionMagicArc"=8, "MotionProfileArc"=10, "Disabled"=15] ("Control Mode")
        n106 = call "Command Drive Distance with Heading Delay.vi"("Turn_Distance"=w314, "Heading"=w313, "Distance"=w312, "Startup"=w311) -> ("Right Wheel"=w308:dbl, "Reinit"=w307:bool, "Left Wheel"=w309:dbl, "Completed"=w310:bool)  [unwired: 4 in]
        n107 = Send Notification(notification=w310, notifier=w315) -> ()  [unwired: 1 in, 2 out]
      }
    }
    "error out" <- w20
    n108 = feedback-in #1(w18) -> ()
    n109 = call <vilib>:"CTRE_Phoenix_MotorControl_Set.vi"("Output"=w21, "Control Mode"=w30, "PhoenixMotorControlDevRef"=w28) -> ()  [unwired: 7 in, 2 out]
    n110 = call <vilib>:"CTRE_Phoenix_MotorControl_Set.vi"("Output"=w22, "Control Mode"=w31, "PhoenixMotorControlDevRef"=w33) -> ()  [unwired: 7 in, 2 out]
  }
